vi "prob_solved.vi"() -> ()   [LabVIEW 2019]
panel:
  out "Waveform Chart 2":dbl(graph)
  out "Waveform Chart":dbl(graph)
  in  "stop":bool
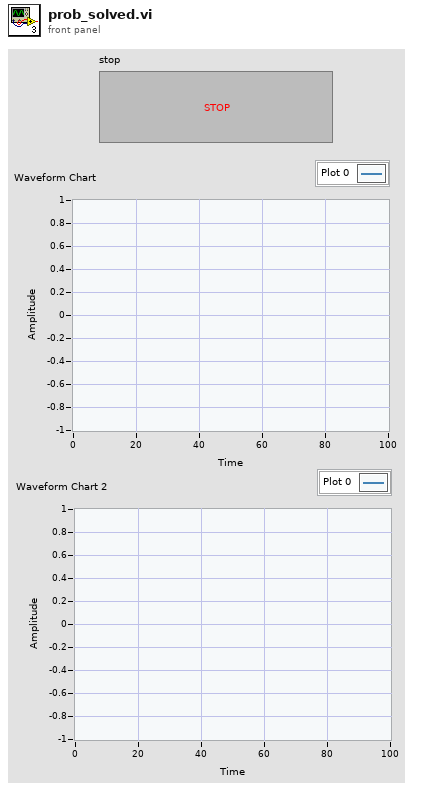
[diagram p1: front panel]
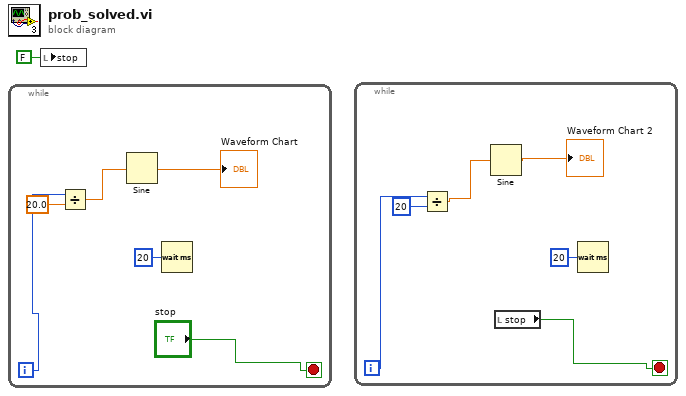
[diagram p0: block diagram]
diagram:
  n1 = while {
    i -> [w5]
    stop <- "stop" stop-if-true
    n2 = Divide(x=w5, y=20.0) -> (x/y=w6:dbl)
    n3 = Sine(x=w6) -> (sin(x)=→"Waveform Chart":dbl)
    n4 = Wait (ms)(milliseconds to wait=u32 20) -> ()  [unwired: 1 out]
  }
  n5 = local write "stop"(FALSE ("stop")) -> ()
  n6 = while {
    i -> [w13]
    stop <- w10 stop-if-true
    n7 = Divide(x=w13, y=20) -> (x/y=w11:dbl)
    n8 = Sine(x=w11) -> (sin(x)=→"Waveform Chart 2":dbl)
    n9 = local read "stop"() -> (w10:bool)
    n10 = Wait (ms)(milliseconds to wait=u32 20) -> ()  [unwired: 1 out]
  }
